vi "Check SQLite Write --Unit Test.vi"(8 "error in":errorcluster, 11 "SQLite Connection":refnum<class "Connection.lvclass">) -> (0 "error out":errorcluster, 3 "Test Result":cluster{"Message":string, "Passed?":bool})   [LabVIEW 2021]
uses:
  <vilib>/drjdpowell/SQLite Library/SQL Connection/Connection.lvclass
  <vilib>/drjdpowell/SQLite Library/SQL Connection/Execute SQL.vi
  <vilib>/drjdpowell/SQLite Library/SQLite.lvlib
panel:
  in  "Expected Column Names":string[](array[string])=["DeviceID", "Name", "Type", "Location"]
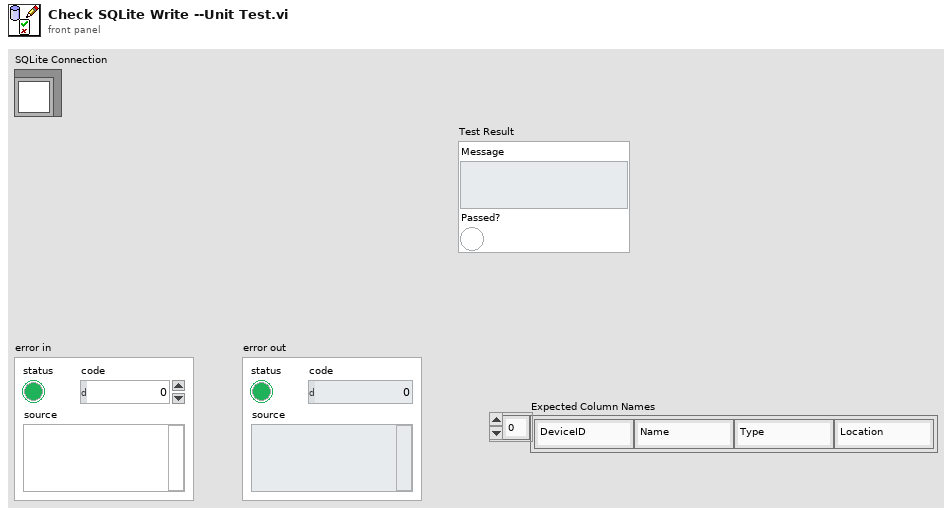
[diagram p1: front panel]
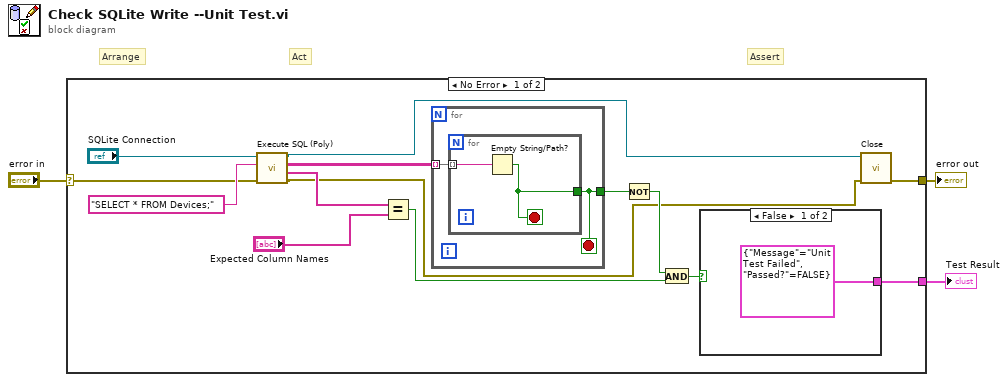
[diagram p0: block diagram]
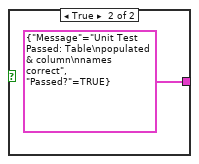
[diagram p2: hidden frame]
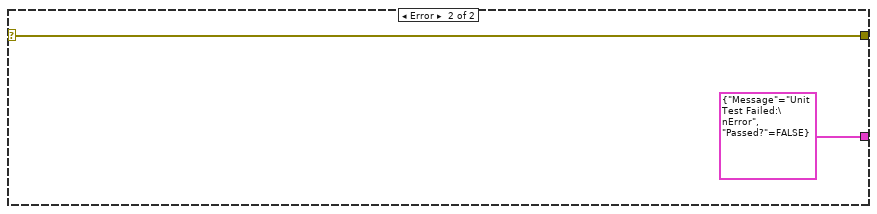
[diagram p3: hidden frame]
diagram:
  # "Assert"
  # "Act"
  # "Arrange"
  n1 = case shown="No Error" "error in" {
    selector: "error in" -> [w14 w25]
    tunnel: [w15 w25] -> w2
    tunnel: [w6 cluster{"Message":string, "Passed?":bool} {"Message"="Unit Test Failed:\nError", "Passed?"=FALSE}] -> w1
    frame No Error {
      n2 = call-poly <vilib>:"Execute SQL (Poly).vi"("error in (no error)"=w14, "SQL"="SELECT * FROM Devices;", "SQLite Connection in"="SQLite Connection") -> ("error out"=w5:errorcluster, "Column Names"=w13:string[], "Result Set"=w11:string[][], "SQLite Connection"=w9:refnum<class "Connection.lvclass">)  [unwired: 5 in]
      n3 = Equal?(x=w13, y="Expected Column Names") -> (x = y?=w4:bool)
      n4 = for {
        tunnel: w11 -> [w21] mode=indexing
        tunnel: [w20] -> w10
        stop <- w20 stop-if-true
        n5 = for {
          tunnel: w21 -> [w23] mode=indexing
          tunnel: [w22] -> w20
          stop <- w22 stop-if-true
          n6 = Empty String/Path?(string/path=w23) -> (empty?=w22:bool)
        }
      }
      n7 = Not(x=w10) -> (.not. x?=w8:bool)
      n8 = And(x=w8, y=w4) -> (x .and. y?=w7:bool)
      n9 = case shown="False" w7 {
        tunnel: [cluster{"Message":string, "Passed?":bool} {"Message"="Unit Test Failed", "Passed?"=FALSE} cluster{"Message":string, "Passed?":bool} {"Message"="Unit Test Passed: Table\npopulated & column\nnames correct", "Passed?"=TRUE}] -> w6
        frame False {
        }
        frame True {
        }
      }
      n10 = call-dynamic "Close.vi"("error in (no error)"=w5, "SQLite Connection in"=w9) -> ("error out"=w15:errorcluster)  [unwired: 9 in]
    }
    frame Error {
    }
  }
  "error out" <- w2
  "Test Result" <- w1
